vi "APC_9049_CAS_loop.vi"(0 "DAQqueues":T1, 1 "error in":errorcluster, 2 "scaled dAQmx task":refnum<k21>) -> ()   [LabVIEW 2020]
doc: "This example demonstrates the procedure required to apply different NI-DAQmx Custom Scales to each virtual channel in a task. A DAQmx Task Property Node (Functions >> NI Measurements >> DAQmx - Data Acquisition >> DAQmx Advanced Task Options) is used to obtain the task's virtual channels. A DAQmx Channel Property Node (Functions >> NI Measurements >> DAQmx - Data Acquisition) is then used to set the custom scale for each virtual channel in the task.\n\nThe \"DAQmx Create Scale\" VI creates a custom scale for each channel in the channel list. *Note, make sure your Minimum and Maximum channel parameters are consistent with the range the scale will create."
uses:
  controls/APC_DAQqueues.ctl
  <vilib>/Platform/TimedLoop/XDataNode/timing_clust.ctl
  <vilib>/Platform/TimedLoop/XDataNode/nitl_modes.ctl
  <vilib>/Platform/TimedLoop/XDataNode/wakeup.ctl
  <vilib>/DAQmx/read.llb/DAQmx Read (Analog 2D DBL NChan NSamp).vi
  <vilib>/DAQmx/miscellaneous.llb/DAQmx Fill In Error Info.vi
  <vilib>/Utility/file.llb/Read Delimited Spreadsheet (DBL).vi
  <vilib>/Platform/TimedLoop/XDataNode/XDataNode.xnode
  <vilib>/Platform/TimedLoop/XDataNode/XDNodeRunTimeDep.lvlib
panel:
  out "9049_EngineSpeed_RPM":dbl
  in  "Sim folder":path=path "/home/lvuser/sim/baseline_fired"
  in  "SIM pressure?":bool
  out "9056 IO":dbl[](array[numeric])
  out "rpm from DAQ":dbl
  out "CAS DAQmx error":errorcluster
  in  "ForceReSync":bool
  in  "AI Graph":bool
  out "Graph time":dbl[][](graph)
  in  "Enque?":bool=TRUE
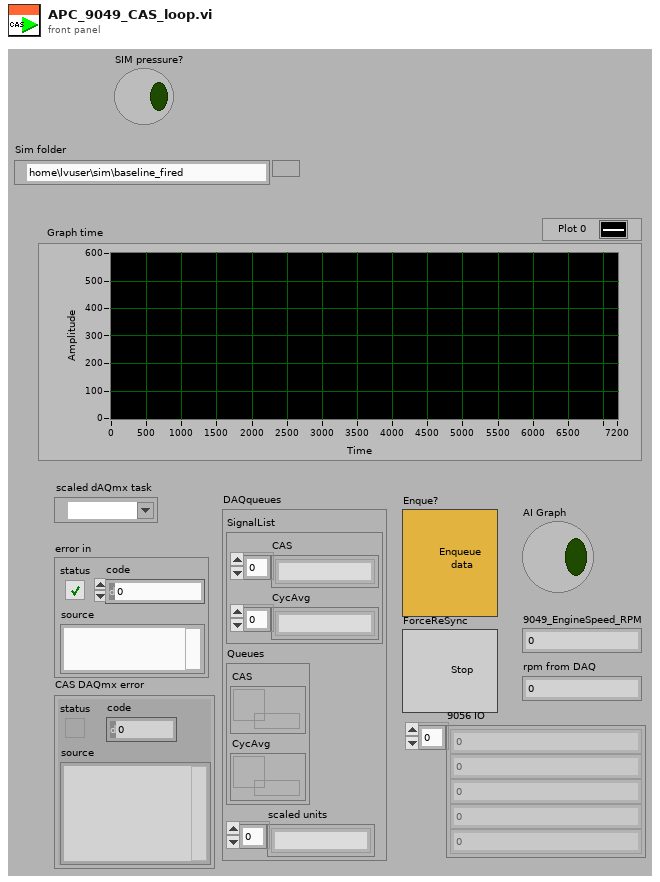
[diagram p1: front panel]
types:
  T1 = typedef "APC_DAQqueues.ctl" = cluster{"SignalList":cluster{"CAS":string[], "CycAvg":string[]}, "Queues":cluster{"CAS":refnum<queue>, "CycAvg":refnum<queue>}, "scaled units":string[]}
  T2 = cluster{"IIR LowPass":cluster{"filter structure":enum32{"IIR 2nd Order", "IIR 4th Order"}, "Reverse Coefficients":dbl[], "Forward Coefficients":dbl[]}, "IIR HighPass":cluster{"filter structure":enum32{"IIR 2nd Order", "IIR 4th Order"}, "Reverse Coefficients":dbl[], "Forward Coefficients":dbl[]}}
  T3 = typedef "APC_CylDaignosticsCluster.ctl" = cluster{"samples for running IMEP std":i32, "MaxDevFromExpectedIMEPError [bar]":dbl, "MaxDevFromExpectedIMEPWarning [bar]":dbl, "MaxDevFromAvgError [bar]":dbl, "MaxDevFromSelfAvgWarning [bar]":dbl, "MaxDevFromSelfAvgError [bar]":dbl, "MaxDevFromAvgWarning [bar]":dbl, "MaxIMEPstdWarning [bar]":dbl, "MaxIMEPstdError [bar]":dbl, "MAPOmaxError [bar/CAD]":dbl, "MAPOmaxWarning [bar/CAD]":dbl, "CA50maxError [CADATDC]":dbl, "CA50maxWarning [CADATDC]":dbl, "MaxPCylMaxError [bar]":dbl, "MaxPCylMaxWarning [bar]":dbl}
  T4 = typedef "XDNodeRunTimeDep.lvlib/timing_clust.ctl" = cluster{"Expected End [f-1]":u64, "Actual End [f-1]":u64, "Finished Late? [f-1]":bool, "Expected End [i-1]":u64, "Actual End [i-1]":u64, "Finished Late? [i-1]":bool, "Expected Start [i]":u64, "Actual Start [i]":u64, "Expected Start [f]":u64, "Actual Start [f]":u64, "Source Name":string, "Structure Name":string, "Period":i64, "Deadline":i64, "Offset":i64, "Start":i64, "Priority":i32, "Timeout":i32, "Mode":T5, "Wakeup Reason":T6, "Error":errorcluster, "Source Type":string, "Secondary Source Type":string, "Global End Time":u64, "Global Start Time":u64, "Frame Duration":u64, "Iteration Duration":u64, "Assigned CPU":i32, "I/O Scan Engine Mode":u32}
  T5 = typedef "XDNodeRunTimeDep.lvlib/nitl_modes.ctl" = enum32{"No Change", "Process missed periods, maintain original phase", "Discard missed periods, maintain original phase", "Process missed periods, ignore original phase", "Discard missed periods, ignore original phase"}
  T6 = typedef "XDNodeRunTimeDep.lvlib/wakeup.ctl" = enum32{"Normal", "Aborted", "Asynchronous wakeup", "Timing source error", "Timed loop error", "Timeout"}
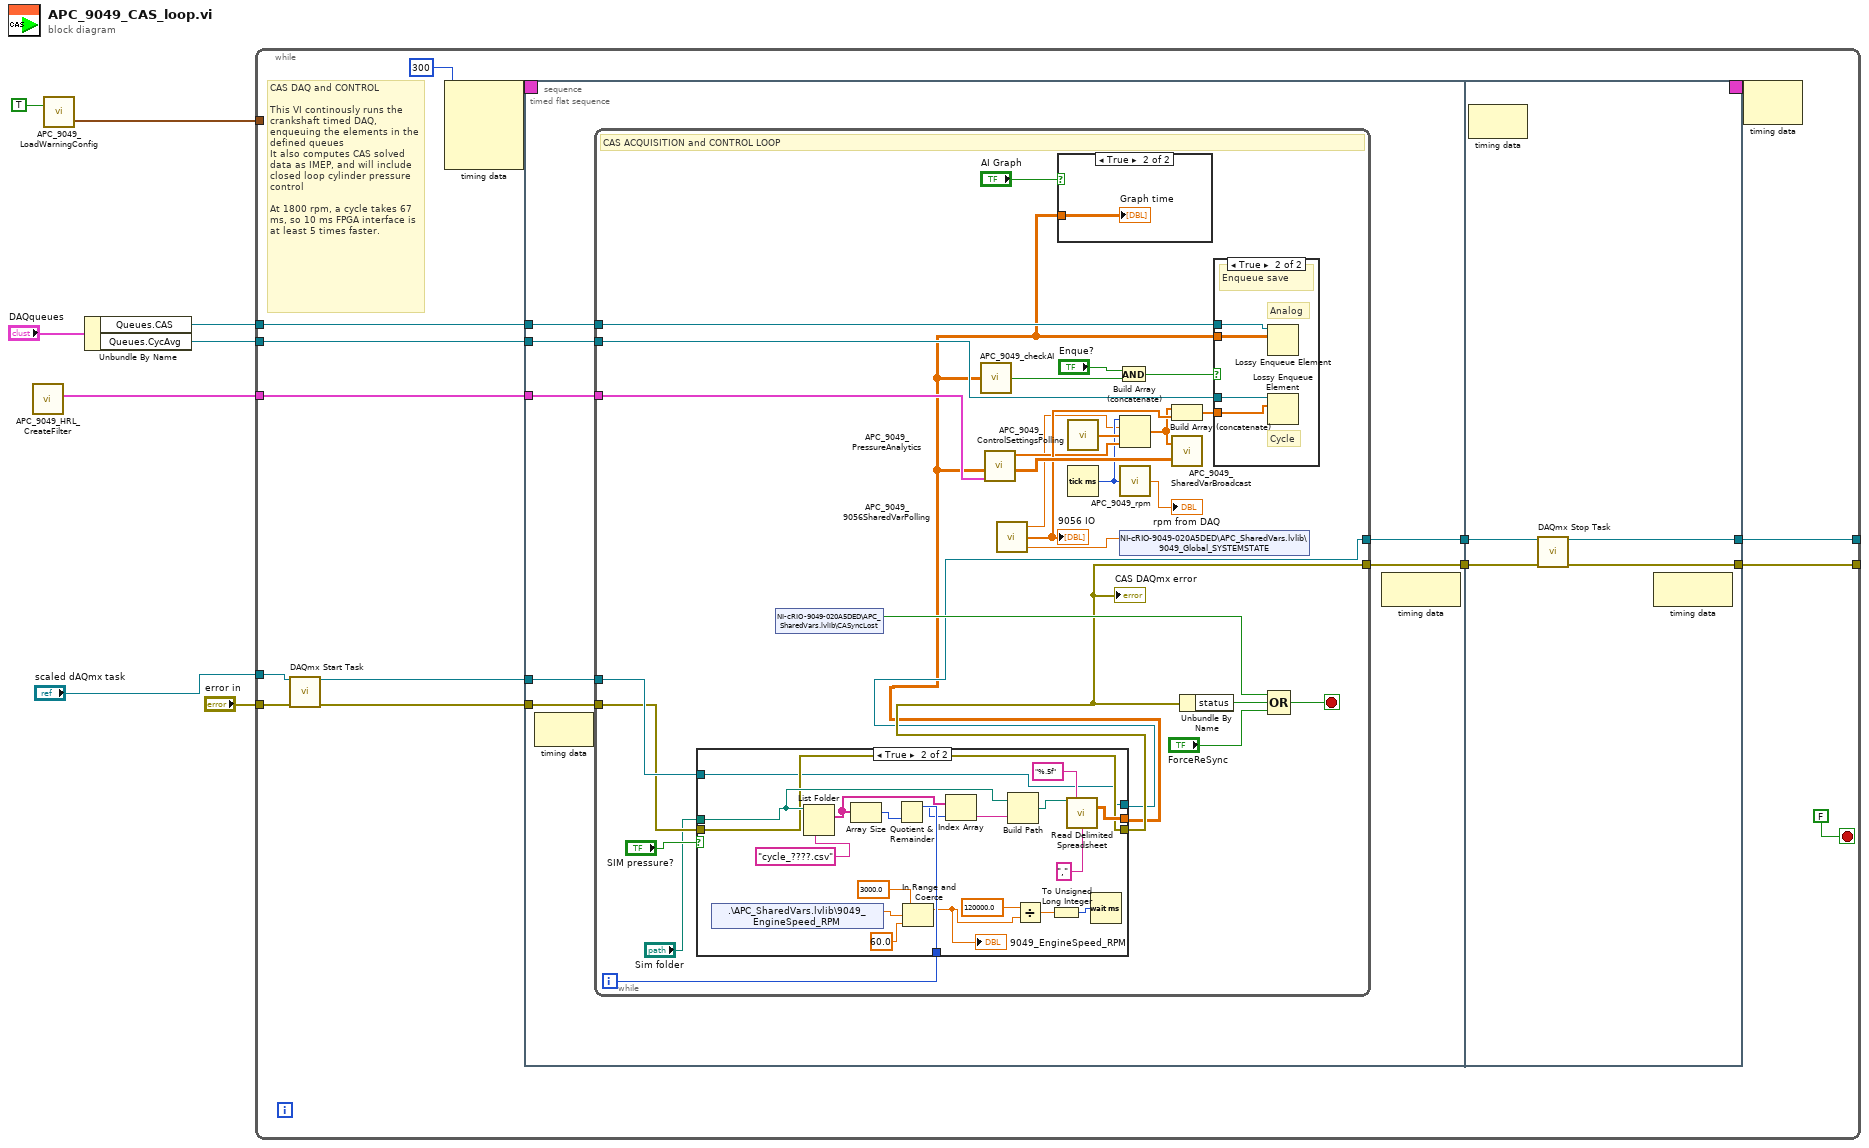
[diagram p0: block diagram]
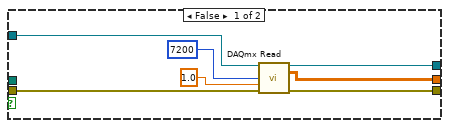
[diagram p2: hidden frame]
diagram:
  n1 = call "APC_9049_HRL_CreateFilter.vi"() -> ("FilterCoefs"=w3:T2)  [unwired: 11 in]
  n2 = call "APC_9049_LoadWarningConfig.vi"("Load?"=TRUE) -> ("CylinderDiagnosticsCluster 2"=w2:T3)  [unwired: 2 in]
  n3 = Unbundle By Name("DAQqueues") -> ("Queues.CAS"=w8:refnum<queue>, "Queues.CycAvg"=w7:refnum<queue>)
  n4 = while {
    tunnel: w8 -> [w18]
    tunnel: w7 -> [w17]
    tunnel: "scaled dAQmx task" -> [w16]
    tunnel: "error in" -> [w15]
    tunnel: [w12] -> _
    tunnel: [w11] -> _
    tunnel: w3 -> [w10]
    tunnel: w2 -> [_]
    stop <- FALSE stop-if-true
    # "CAS DAQ and CONTROL\n\nThis VI continously runs the crankshaft timed DAQ, enqueuing the elements in the defined queues \nIt also computes CAS solved data as IMEP, and will include closed loop cylinder pressure control\n\nAt 1800 rpm, a cycle takes 67 ms, so 10 ms FPGA interface is at least 5 times faster."
    n5 = call <vilib>:"DAQmx Start Task.vi"("task/channels in"=w16, "error in"=w15) -> ("task out"=w14:refnum<k21>, "error out"=w13:errorcluster)  [unwired: 12 in]
    n6 = node-c288(300 ("Priority")) -> (w21:T4)  [unwired: 3 in]
    n7 = timed-sequence {
      timing: w21 -> [_]
      timing-out: [_] -> w20
      tunnel: w14 -> [w30]
      tunnel: w13 -> [w29]
      tunnel: w18 -> [w28]
      tunnel: w17 -> [w27]
      tunnel: [w24] -> w12
      tunnel: [w23] -> w11
      tunnel: w10 -> [w22]
      n8 = timed-flat-sequence {
        tunnel: w30 -> [w37]
        tunnel: w29 -> [w36]
        tunnel: w28 -> [w33]
        tunnel: w27 -> [w32]
        tunnel: [w35] -> w26
        tunnel: [w34] -> w25
        tunnel: w22 -> [w31]
        tunnel: w26 -> [w104]
        tunnel: w25 -> [w103]
        tunnel: [w101] -> w24
        tunnel: [w102] -> w23
        frame #0 {
          n9 = node-c288() -> ()  [unwired: 1 in, 1 out]
          n10 = while {
            tunnel: w37 -> [w47]
            tunnel: w36 -> [w46]
            tunnel: [w44] -> w35
            tunnel: [w45] -> w34
            tunnel: w33 -> [w67]
            tunnel: w32 -> [w66]
            tunnel: w31 -> [w53]
            i -> [w40]
            stop <- w62 stop-if-true
            # "CAS ACQUISITION and CONTROL LOOP"
            n11 = case shown="True" "SIM pressure?" {
              tunnel: w47 -> [w73 w83]
              tunnel: w46 -> [w72 w84]
              tunnel: [w71 w84] -> w45
              tunnel: [w70 w83] -> w44
              tunnel: [w69 w85] -> w43
              tunnel: "Sim folder" -> [_ w87]
              tunnel: w40 -> [_ w91]
              frame False {
                n12 = call-poly <vilib>:"DAQmx Read.vi"("task/channels in"=w73, "number of samples per channel"=7200, "timeout"=1.0, "error in"=w72) -> ("task out"=w70:refnum<k21>, "data"=w69:dbl[][], "error out"=w71:errorcluster)  [unwired: 9 in]
              }
              frame True {
                n13 = shared-variable ".\\APC_SharedVars.lvlib\\9049_EngineSpeed_RPM"() -> (w79:dbl)  [unwired: 1 in, 1 out]
                n14 = List Folder(path=w87, pattern="cycle_????.csv") -> (filenames=w89:string[])  [unwired: 2 in, 3 out]
                n15 = Array Size(array=w89) -> (size(s)=w92:i32)
                n16 = Quotient & Remainder(x=w91, y=w92) -> (x-y*floor(x/y)=w90:i32)  [unwired: 1 out]
                n17 = In Range and Coerce(upper limit=3000.0, x=w79, lower limit=60.0) -> (coerced(x)=w76:dbl)  [unwired: 1 out]
                "9049_EngineSpeed_RPM" <- w76
                n18 = Index Array(array=w89, index=w90) -> (element=w88:string)
                n19 = Build Path(base path=w87, name or relative path=w88) -> (appended path=w86:path)
                n20 = Divide(x=120000.0, y=w76) -> (x/y=w81:dbl)
                n21 = To Unsigned Long Integer(number=w81) -> (unsigned 32bit integer=w80:u32)
                n22 = call-poly <vilib>:"Read Delimited Spreadsheet.vi"("file path (dialog if empty)"=w86, "format (%.3f)"="%.5f", "delimiter (\\t)"="," ("delimiter (\\t)")) -> ("all rows"=w85:dbl[][])  [unwired: 7 in, 5 out]
                n23 = Wait (ms)(milliseconds to wait=w80) -> ()  [unwired: 1 out]
              }
            }
            "CAS DAQmx error" <- w45
            n24 = shared-variable "NI-cRIO-9049-020A5DED\\APC_SharedVars.lvlib\\CASyncLost"() -> (w63:bool)  [unwired: 1 in, 1 out]
            n25 = call "APC_9049_checkAI.vi"("AIdata [bar]"=w43) -> ("x = y?"=w52:bool)
            n26 = call "APC_9049_PressureAnalytics.vi"("FilterCoefs"=w53, "AIdata [bar]"=w43) -> ("SyncCylPres [bar]"=w61:dbl[][], "9049_CalculatedVariablesRaster"=w56:dbl[])  [unwired: 4 in]
            n27 = call "APC_9049_9056SharedVarPolling.vi"() -> ("TimeStamp9056"=w49:dbl, "9056 IO"=w59:dbl[], "SystemState"=w48:dbl)  [unwired: 1 in, 1 out]
            "9056 IO" <- w59
            n28 = case shown="True" "AI Graph" {
              tunnel: w43 -> [_ w96]
              frame False {
              }
              frame True {
                "Graph time" <- w96
              }
            }
            n29 = call "APC_9049_ControlSettingsPolling.vi"() -> ("9049_ControlSettings"=w57:dbl[])
            n30 = Tick Count (ms)() -> (millisecond timer value=w50:u32)
            n31 = And(x="Enque?", y=w52) -> (x .and. y?=w54:bool)
            n32 = Build Array (concatenate)(w50, w49, w57, w56) -> (w58:dbl[])
            n33 = call "APC_9049_rpm.vi"("millisecond timer value"=w50) -> ("rpm from DAQ"=→"rpm from DAQ":dbl)
            n34 = shared-variable "NI-cRIO-9049-020A5DED\\APC_SharedVars.lvlib\\9049_Global_SYSTEMSTATE"(w48) -> ()  [unwired: 1 in, 1 out]
            n35 = Build Array (concatenate)(w58, w59) -> (w60:dbl[])
            n36 = call "APC_9049_SharedVarBroadcast.vi"("SyncCylPres [bar]"=w61, "9049_MeasAndCalc"=w58) -> ()  [unwired: 1 in]
            n37 = Unbundle By Name(w45) -> ("status"=w64:bool)
            n38 = case shown="True" w54 {
              tunnel: w43 -> [_ w100]
              tunnel: w67 -> [_ w99]
              tunnel: w66 -> [_ w98]
              tunnel: w60 -> [_ w97]
              frame False {
              }
              frame True {
                # "Analog"
                # "Cycle"
                # "Enqueue save"
                n39 = Lossy Enqueue Element(queue=w99, element=w100) -> ()  [unwired: 1 in, 4 out]
                n40 = Lossy Enqueue Element(queue=w98, element=w97) -> ()  [unwired: 1 in, 4 out]
              }
            }
            n41 = Compound Arithmetic op=OR(w63, w64, "ForceReSync") -> (w62:bool)
          }
          n42 = node-c288() -> ()  [unwired: 1 in, 1 out]
        }
        frame #1 {
          n43 = node-c288() -> ()  [unwired: 1 in, 1 out]
          n44 = call <vilib>:"DAQmx Stop Task.vi"("task/channels in"=w104, "error in"=w103) -> ("task out"=w101:refnum<k21>, "error out"=w102:errorcluster)  [unwired: 12 in]
          n45 = node-c288() -> ()  [unwired: 1 in, 1 out]
        }
      }
    }
    n46 = node-c288(w20) -> ()  [unwired: 1 out]
  }
